vi "Video Player.vi"() -> ()   [LabVIEW 2015]
uses:
  <vilib>/vision/Avi.llb/IMAQ AVI2 Codec Path.ctl
panel:
  out "Frame Data":T1
  out "Image Type":T2 items=["Grayscale (U8)", "Grayscale (I16)", "Grayscale (SGL)", "Complex (CSG)", "RGB (U32)", "HSL (U32)", "RGB (U64)", "Grayscale (U16)"]
  out "Number of Frames":u32
  in  "File Path":path=path "D:/Eye Video.avi"
  out "Image Out":T3(plugin-control)
  out "error out":errorcluster
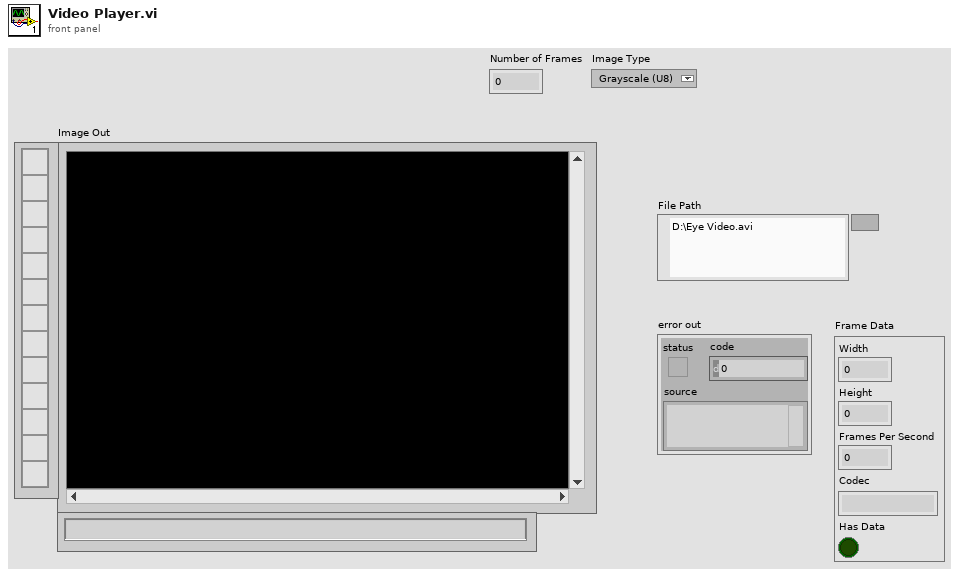
[diagram p1: front panel]
types:
  T1 = cluster{"Width":u32, "Height":u32, "Frames Per Second":u32, "Codec":string, "Has Data":bool}
  T2 = typedef "Image Type" = u32
  T3 = typedef "IMAQ Image.ctl" = refnum<image>
  T4 = typedef "IMAQ AVI2 Codec Path.ctl" = u32
  T5 = typedef "IMAQ AVI2 Refnum.ctl" = refnum<k20>
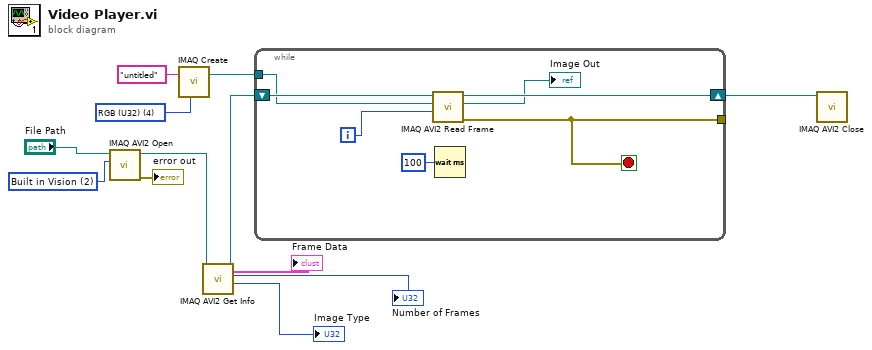
[diagram p0: block diagram]
diagram:
  w7 = T2 4 items=["Grayscale (U8)", "Grayscale (I16)", "Grayscale (SGL)", "Complex (CSG)", "RGB (U32)", "HSL (U32)", "RGB (U64)", "Grayscale (U16)"] ("Image Type")
  w12 = T4 2 items=["Default", "System", "Built in Vision"] ("Codec Source")
  n1 = call "IMAQ AVI2 Open"("Codec Source"=w12, "AVI File Path"="File Path") -> ("error out"=→"error out":errorcluster, "AVI Refnum"=w5:T5)  [unwired: 8 in]
  n2 = call "IMAQ Create"("Image Name"="untitled", "Image Type"=w7) -> ("New Image"=w9:T3)  [unwired: 3 in, 1 out]
  n3 = call "IMAQ AVI2 Get Info"("AVI Refnum"=w5) -> ("Image Type"=→"Image Type":T2, "Number of Frames"=→"Number of Frames":u32, "AVI Refnum (duplicate)"=w4:T5, "Frame Data"=→"Frame Data":T1)  [unwired: 6 in, 1 out]
  n4 = while {
    shift-right: [w17] -> w8
    shift-left: w4 -> [w19]
    tunnel: [w13] -> _
    tunnel: w9 -> [w18]
    i -> [w16]
    stop <- w13 stop-if-true
    n5 = call "IMAQ AVI2 Read Frame"("Frame Number"=w16, "Image"=w18, "AVI Refnum"=w19) -> ("error out"=w13:errorcluster, "Image Out"=→"Image Out":T3, "AVI Refnum (duplicate)"=w17:T5)  [unwired: 6 in]
    n6 = Wait (ms)(milliseconds to wait=u32 100) -> ()  [unwired: 1 out]
  }
  n7 = call "IMAQ AVI2 Close"("AVI Refnum"=w8) -> ()  [unwired: 10 in, 1 out]
